vi "Snapshot Viewer.vi"() -> ()   [LabVIEW 2018]
uses:
  <userlib>/Jet Engineering/JET_QSM/Code/Private/JET_QSM - Add State [String API].vi
  <userlib>/Jet Engineering/JET_QSM/Code/Private/JET_QSM_InvalidOption STYP.ctl
  Private/Status STYP.ctl
  Classes/Video File/Video File.lvclass
  Classes/Video Frame/Video Frame.lvclass
  <vilib>/vision/Image Controls.llb/IMAQ Image.ctl
  Classes/Message/Message.lvclass
  Classes/Depth Data Message/Depth Data Message.lvclass
  Classes/STOP Message/STOP.lvclass
  <vilib>/Utility/Data Type/NI_Data Type.lvlib
  C:/Users/aaron.jencks/Documents/GitHub/emerson_seed_object_detection/LabVIEW/Projects/Paul's Video Viewer/Classes/Message/Message.lvclass
  Shared/Roughness Parameters STYP.ctl
panel:
  in  "Clear?":bool
  out "Ready?":bool
  out "Saved Indices":u32[](array[numeric])
  in  "Keep?":bool
  in  "stop":bool
  out "File Opened?":bool
  out "Frame Count":u32
  in  "Frame Index":u32
  out "Roughness Parameters":T1
  in  "Path":path
  out "Image":T2(plugin-control)
  out "Recent states before Error (with tick counts) 2":string="0.167 sec ago: VI Initialize\n0.167 sec ago: Window Open\n0.110 sec ago: Control Update\n0.110 sec ago: Indicator Update\n0.000 sec ago: Error Handler\r\n"
  out "error out":errorcluster
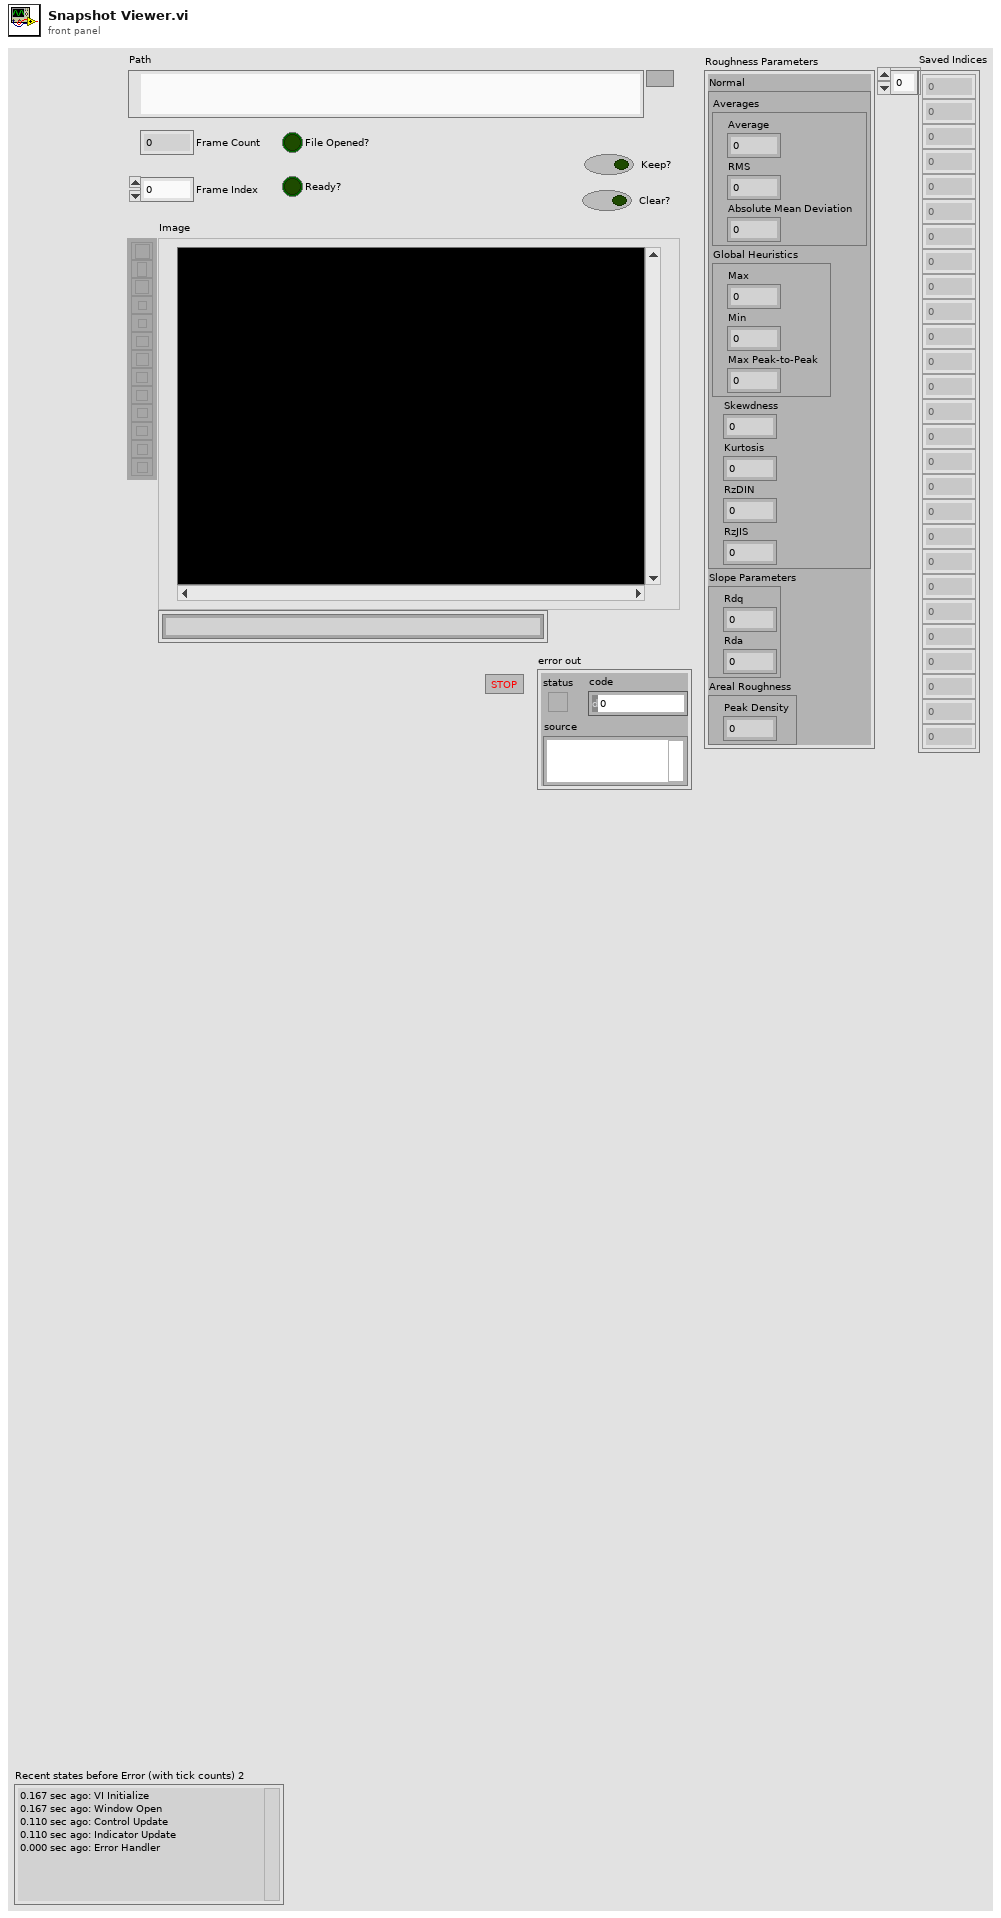
[diagram p1: front panel]
types:
  T1 = typedef "Roughness Parameters STYP.ctl" = cluster{"Normal":cluster{"Averages":cluster{"Average":dbl, "RMS":dbl, "Absolute Mean Deviation":dbl}, "Global Heuristics":cluster{"Max":dbl, "Min":dbl, "Max Peak-to-Peak":dbl}, "Skewdness":dbl, "Kurtosis":dbl, "RzDIN":dbl, "RzJIS":dbl}, "Slope Parameters":cluster{"Rdq":dbl, "Rda":dbl}, "Areal Roughness":cluster{"Peak Density":dbl}}
  T2 = typedef "IMAQ Image.ctl" = refnum<image>
  T3 = typedef "Status STYP.ctl" = cluster{"VI":cluster{"error":errorcluster, "isExiting?":bool}, "UserLoggedIn?":bool, "Frame Index":u32, "Video File":refnum<class "Video File.lvclass">, "Current Frame":refnum<class "Video Frame.lvclass">, "Image Placeholder":T2, "data log queue":refnum<queue>, "stop queue":refnum<queue>, "Saved Indices":u32[], "ready queue":refnum<queue>}
  T4 = typedef "JET_QSM_InvalidOption STYP.ctl" = enum16{"Ignore", "Dialog", "Error"}
  T5 = typedef "JET_QSM_Refnum STYP.ctl" = cluster{"state":cluster{"queue":refnum<queue>, "idle":string, "error":string, "STOP":string}, "debug":cluster{"enabled?":bool, "queue":refnum<queue>}, "Invalid.option":T4, "QSM.Name":string}
  T6 = enum32{"invalid app kind", "Development System", "Run Time System", "Student Edition", "Embedded LabVIEW", "Evaluation", "Custom"}
  T7 = typedef "JET_QSM_Element STYP.ctl" = cluster{"state":string, "data":variant, "comment":string}
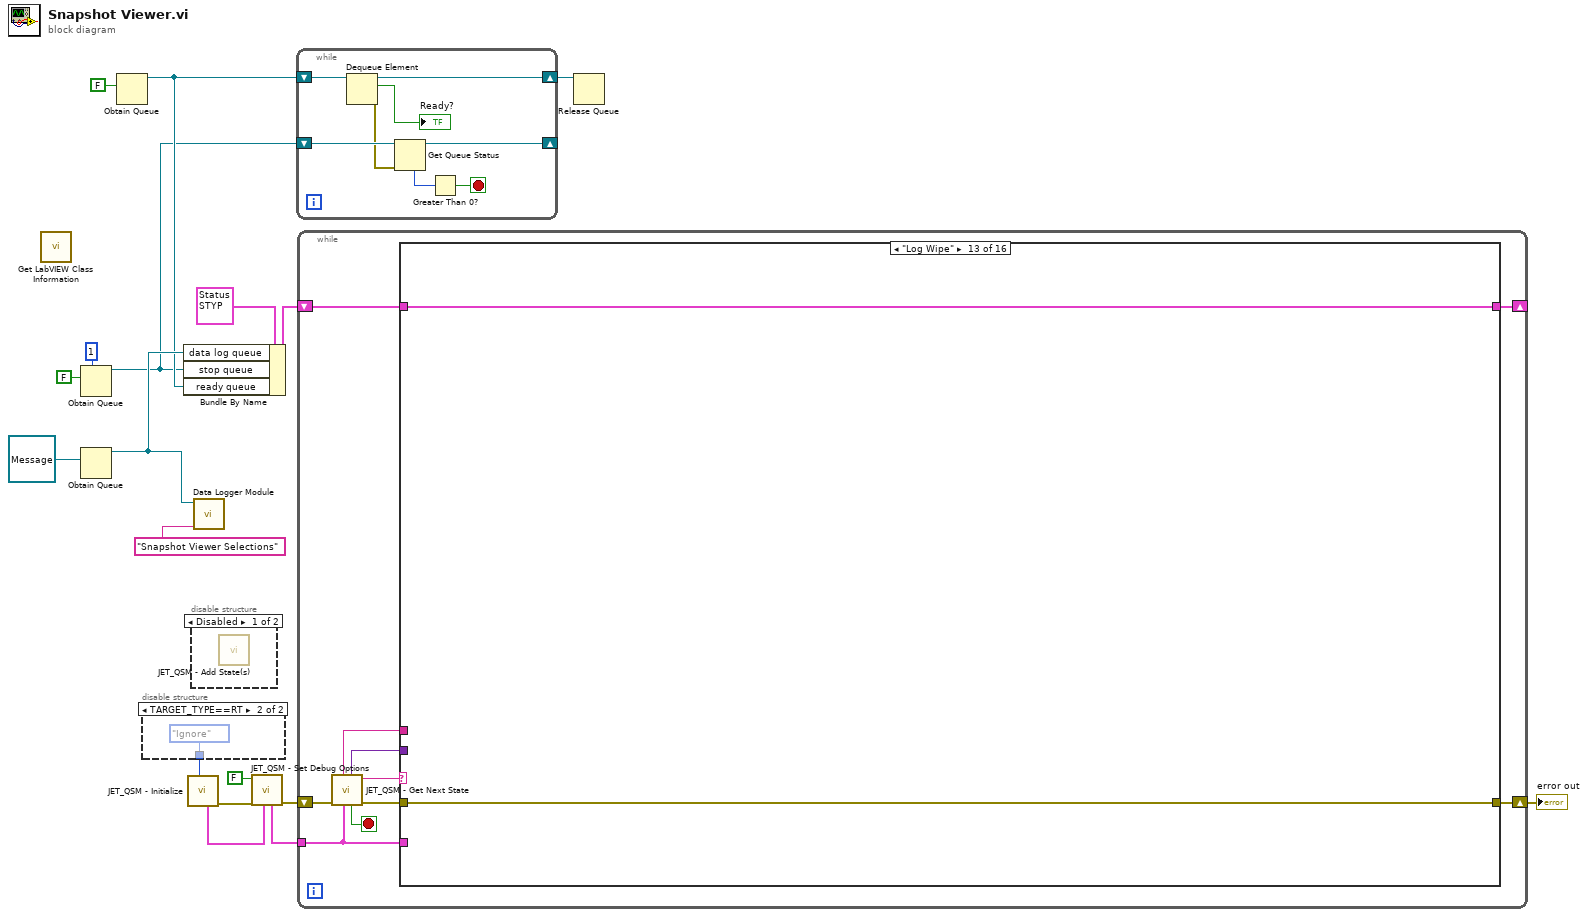
[diagram p0: block diagram]
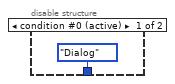
[diagram p2: hidden frame]
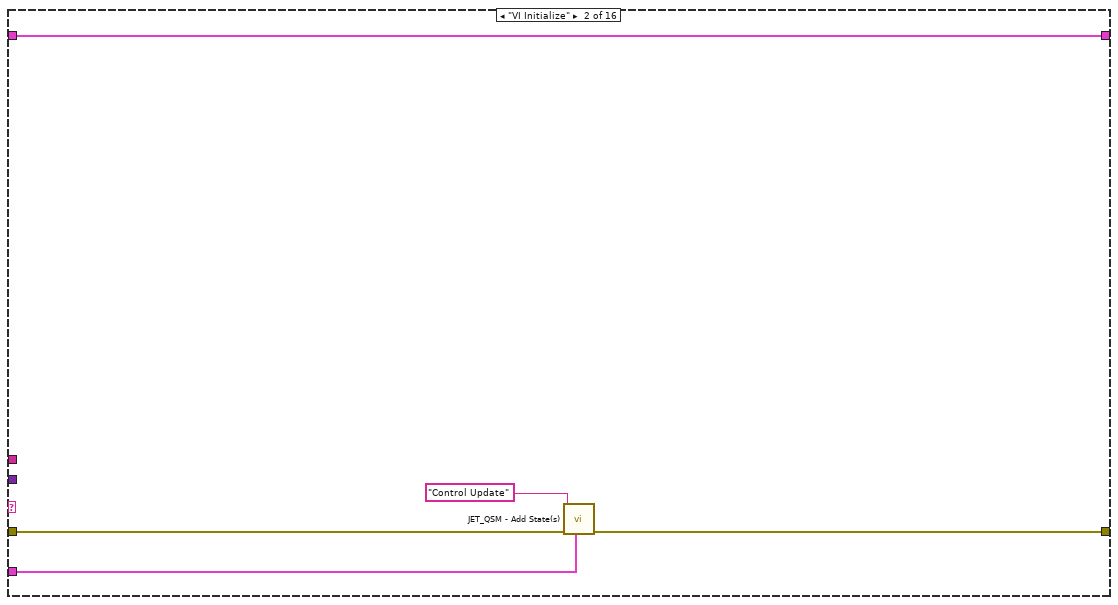
[diagram p5: hidden frame]
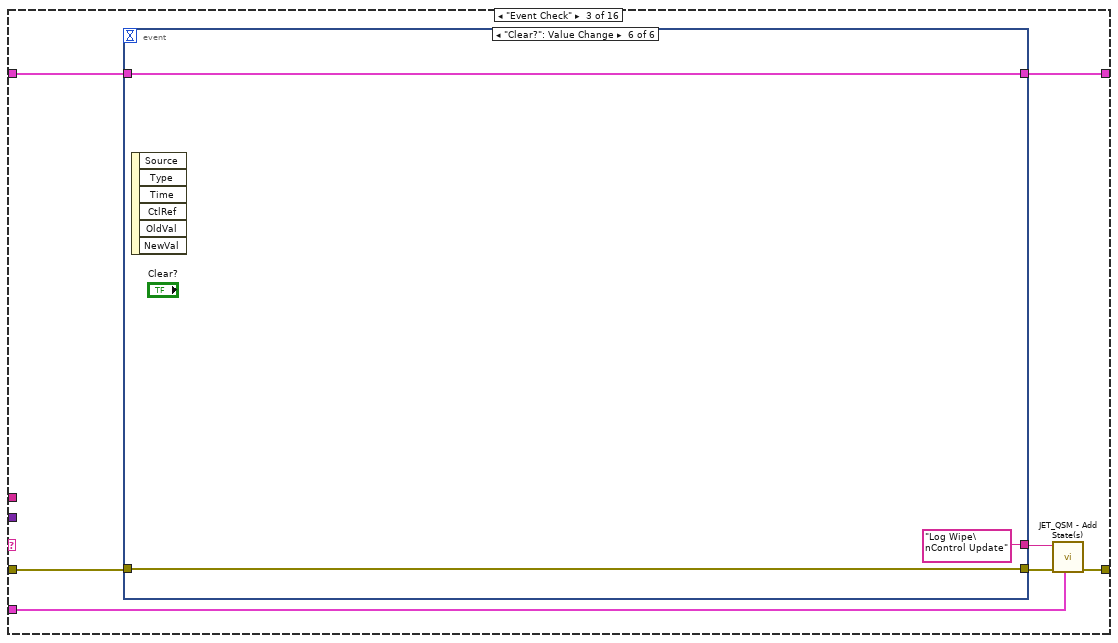
[diagram p6: hidden frame]
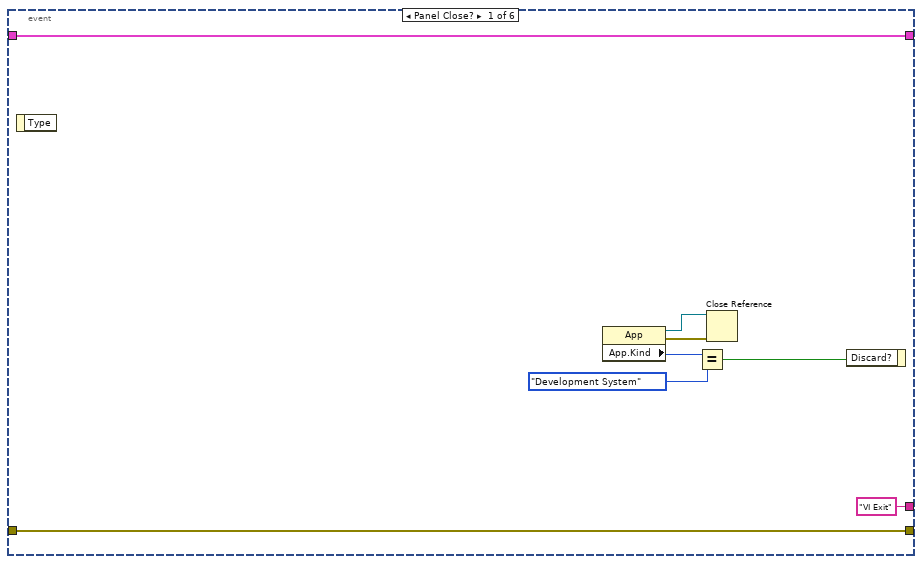
[diagram p7: hidden frame]
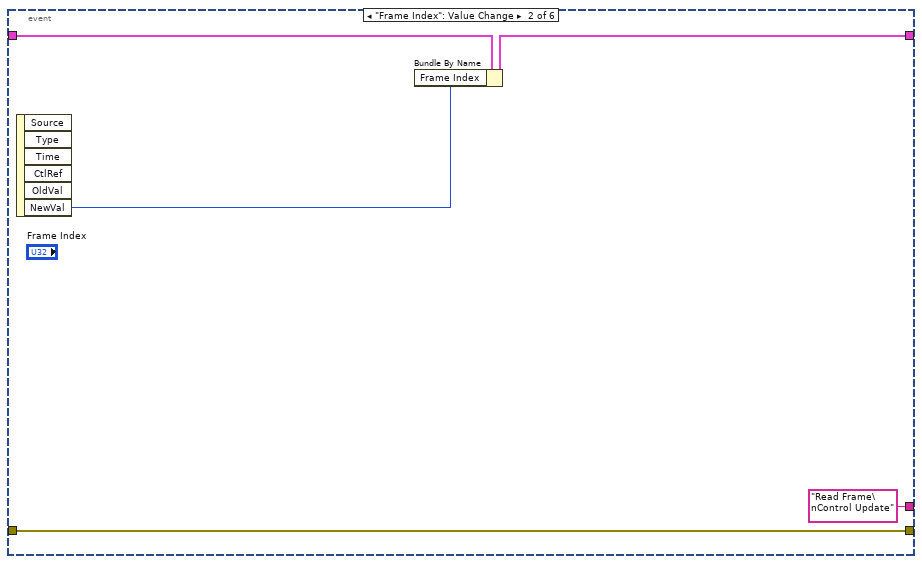
[diagram p8: hidden frame]
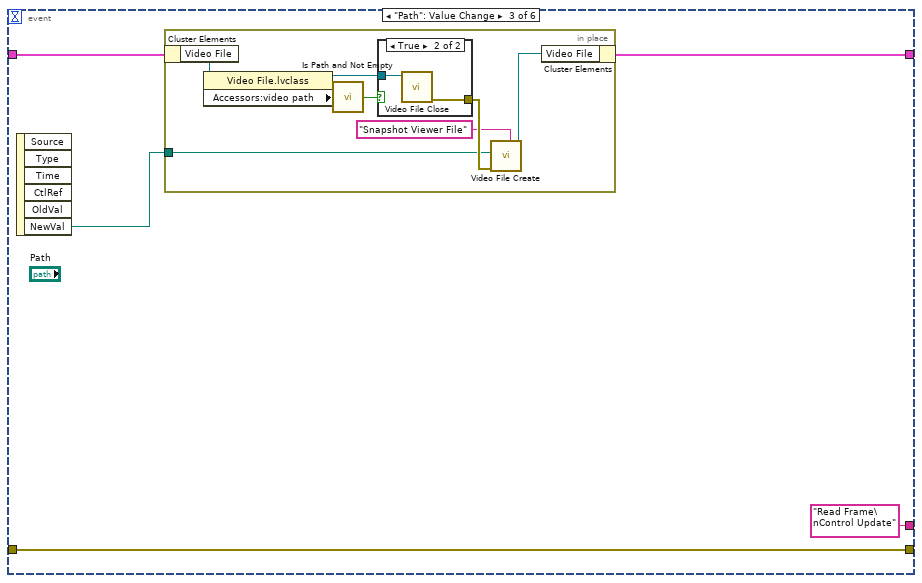
[diagram p9: hidden frame]
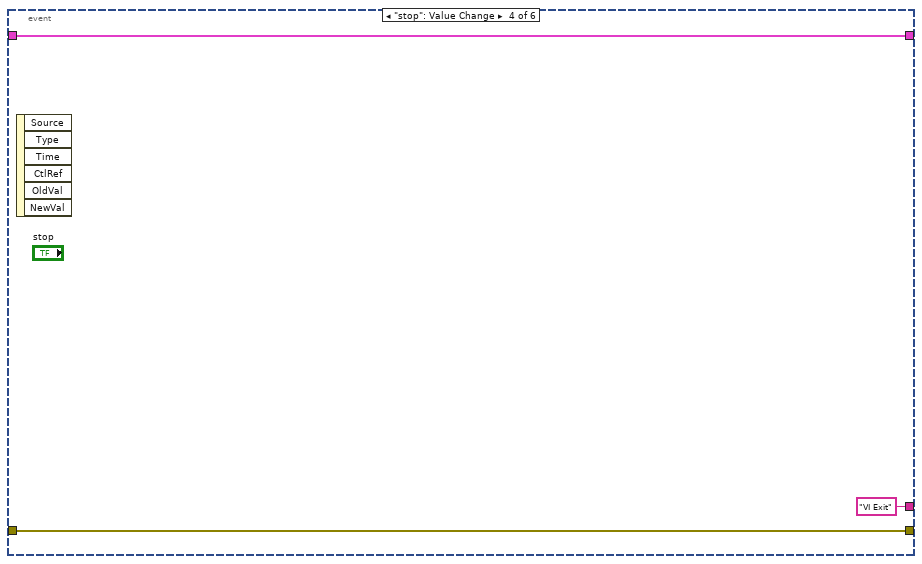
[diagram p11: hidden frame]
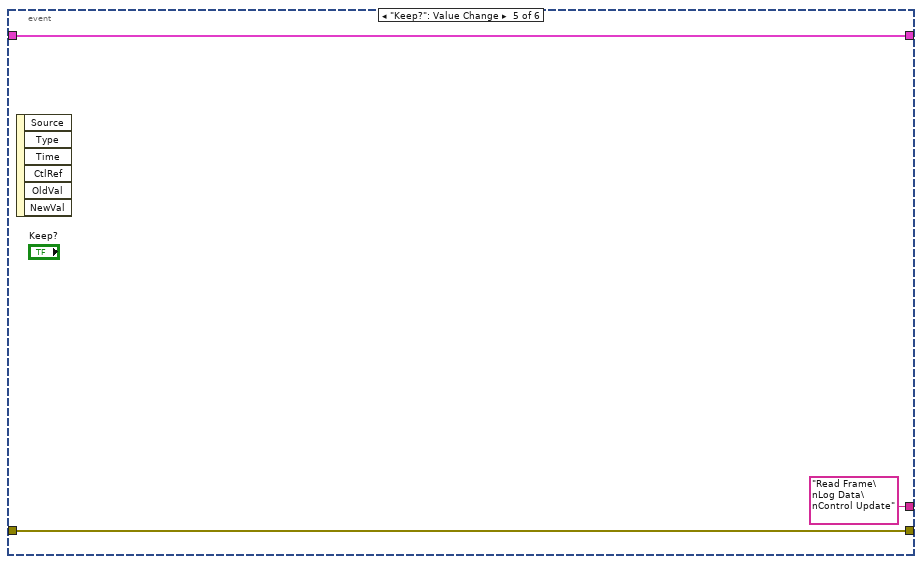
[diagram p12: hidden frame]
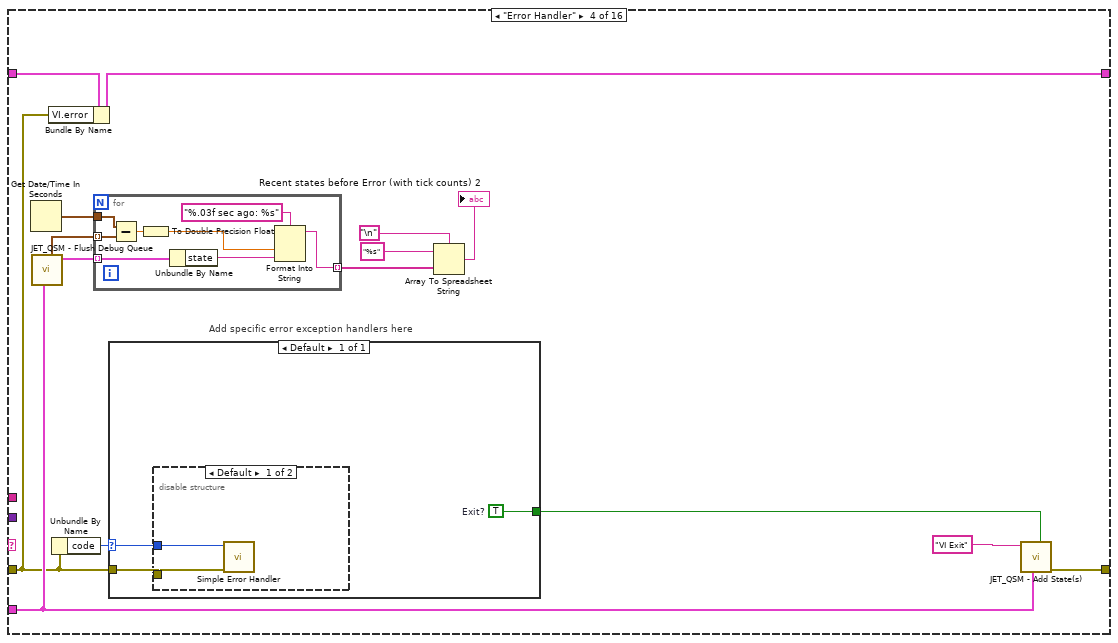
[diagram p13: hidden frame]
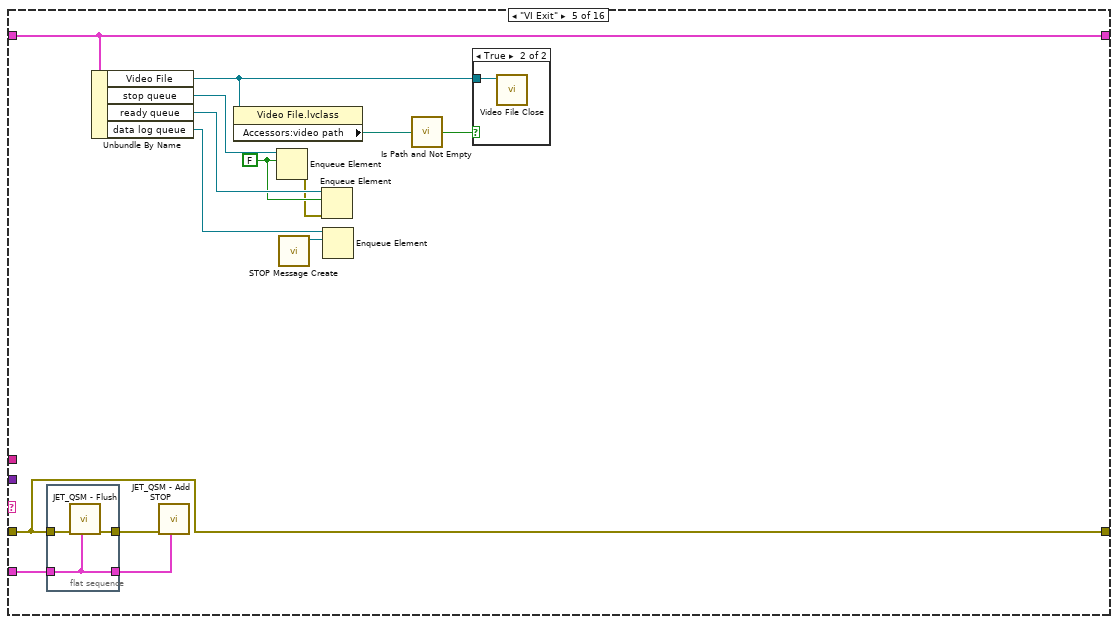
[diagram p15: hidden frame]
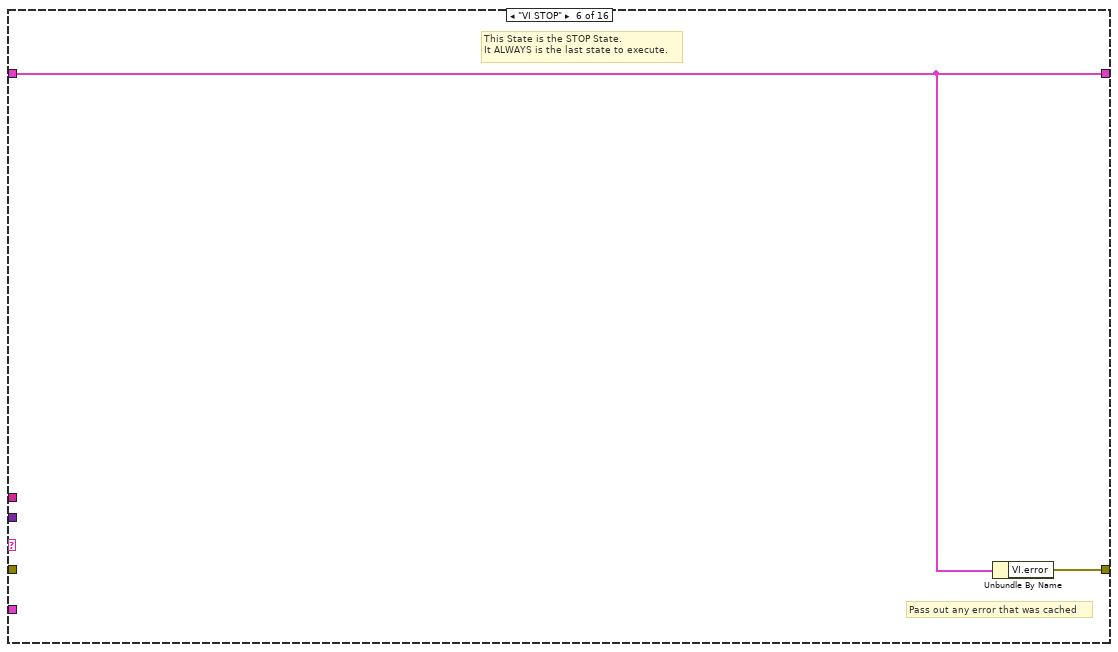
[diagram p17: hidden frame]
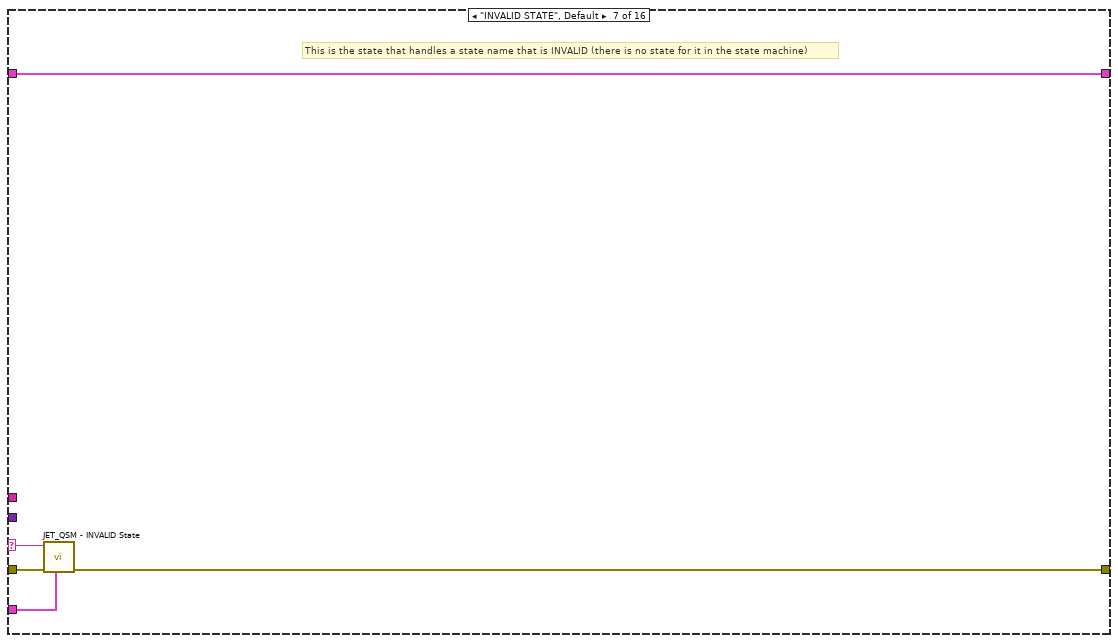
[diagram p18: hidden frame]
diagram:
  n1 = call <vilib>:"Get LabVIEW Class Information.vi"() -> ()  [unwired: 9 in, 3 out]
  n2 = Obtain Queue(max queue size (-1, unlimited)=1, element data type=FALSE) -> (queue out=w3:refnum<queue>)  [unwired: 3 in, 2 out]
  n3 = Obtain Queue(element data type=refnum<class "Message.lvclass"> refnum ("Message.lvclass")) -> (queue out=w7:refnum<queue>)  [unwired: 4 in, 2 out]
  n4 = Obtain Queue(element data type=FALSE) -> (queue out=w4:refnum<queue>)  [unwired: 4 in, 2 out]
  n5 = disable-structure shown="TARGET_TYPE==RT" {
    disable-tunnel: [JET_QSM_InvalidOption_STYP."Dialog" ("invalid state action (Dialog)") JET_QSM_InvalidOption_STYP."Ignore" ("invalid state action (Dialog)")] -> w18
    frame condition #0 (active) {
    }
    frame condition #1 {
    }
  }
  n6 = Bundle By Name(cluster=T3 {"VI"={"error"={"status"=FALSE, "code"=0, "source"=""}, "isExiting?"=FALSE}, "UserLoggedIn?"=FALSE, "Frame Index"=0, "Video File"=refnum, "Current Frame"=refnum, "Image Placeholder"=refnum, "data log queue"=refnum, "stop queue"=refnum, "Saved Indices"=[], "ready queue"=refnum} ("Status"), "data log queue"=w7, "stop queue"=w3, "ready queue"=w4) -> (w8:T3)
  n7 = call <userlib>:"JET_QSM - Initialize.vi"("invalid state action (Dialog)"=w18) -> ("error out"=w12:errorcluster, "Jet_QSM refnum"=w15:T5)  [unwired: 9 in]
  n8 = disable-structure shown="Disabled" {
    frame Disabled {
      n9 = call-poly <userlib>:"JET_QSM - Add State(s).vi"() -> ()  [unwired: 11 in, 1 out]
    }
    frame Enabled {
    }
  }
  n10 = call "Data Logger Module.vi"("Identifier"="Snapshot Viewer Selections", "Message queue"=w7) -> ()  [unwired: 10 in]
  n11 = call <userlib>:"JET_QSM - Set Debug Options.vi"("Jet_QSM refnum"=w15, "error in (no error)"=w12, "debug.enabled? (F)"=FALSE) -> ("error out"=w13:errorcluster, "Jet_QSM ref"=w14:T5)  [unwired: 7 in]
  n12 = while {
    shift-right: [w26] -> w2
    shift-left: w4 -> [w28]
    shift-right: [w22] -> _
    shift-left: w3 -> [w25]
    stop <- w23 stop-if-true
    n13 = Dequeue Element(queue=w28) -> (queue out=w26:refnum<queue>, element=→"Ready?":bool, error out=w21:errorcluster)  [unwired: 2 in, 1 out]
    n14 = Get Queue Status(queue=w25, error in (no error)=w21) -> (queue out=w22:refnum<queue>, # elements in queue=w24:i32)  [unwired: 1 in, 6 out]
    n15 = Greater Than 0?(x=w24) -> (x > 0?=w23:bool)
  }
  n16 = while {
    tunnel: w14 -> [w34]
    shift-right: [w32] -> _
    shift-left: w8 -> [w33]
    shift-right: [w31] -> w17
    shift-left: w13 -> [w38]
    stop <- w35 stop-if-true
    n17 = call <userlib>:"JET_QSM - Get Next State.vi"("Jet_QSM refnum"=w34, "error in (no error)"=w38) -> ("error out"=w37:errorcluster, "state"=w36:string, "Stop Loop?"=w35:bool, "state data"=w30:variant, "state comment"=w29:string)  [unwired: 5 in]
    n18 = case shown="\"Log Wipe\"" w36 {
      selector: w36 -> [_ _ _ _ _ _ w140 _ _ _ _ _ _ _ _ _]
      tunnel: w37 -> [w39 w43 w52 w91 w131 _ w141 w143 w145 w147 w165 w179 w193 w195 w204 w219]
      tunnel: w34 -> [_ w44 w51 w96 w129 _ w139 _ _ _ _ _ _ _ w205 _]
      tunnel: w33 -> [w40 w45 w47 w92 w127 w136 w142 w144 w146 w148 w163 w174 w194 w196 w202 w218]
      tunnel: [w40 w45 w46 w90 w127 w136 w142 w144 w146 w148 w161 w172 w194 w196 w202 w218] -> w32
      tunnel: [w39 w42 w49 w97 w131 w137 w138 w143 w145 w147 w165 w179 w193 w195 w203 w219] -> w31
      tunnel: w30 -> [_ _ _ _ _ _ _ _ _ _ _ _ _ _ _ _]
      tunnel: w29 -> [_ _ _ _ _ _ _ _ _ _ _ _ _ _ _ _]
      frame "------ Standard States ------" {
        # "Standard States are required states for a JET_QSM State Machine\n\nTheir names may be changed; use the Initialize function to specify the new names"
        # "This is a section header; the state is never expected to execute"
      }
      frame "VI Initialize" {
        n19 = call-poly <userlib>:"JET_QSM - Add State(s).vi"("Jet_QSM refnum"=w44, "error in (no error)"=w43, "state(s)"="Control Update") -> ("error out"=w42:errorcluster)  [unwired: 8 in]
      }
      frame "Event Check" {
        n20 = event shown="[5] \"Clear?\": Value Change" {
          selector: _ -> [_ _ _ _ _ _]
          dyn-events: _ -> [_ _ _ _ _ _]
          timeout: _ -> [_ _ _ _ _ _]
          tunnel: w52 -> [w54 w65 w70 w82 w85 w88]
          tunnel: ["VI Exit" ("state(s)") "Read Frame\nControl Update" ("state(s)") "Read Frame\nControl Update" ("state(s)") "VI Exit" ("state(s)") "Read Frame\nLog Data\nControl Update" ("state(s)") "Log Wipe\nControl Update" ("state(s)")] -> w50
          tunnel: [w54 w65 w70 w82 w85 w88] -> w48
          tunnel: w47 -> [w53 w63 w68 w83 w86 w89]
          tunnel: [w53 w61 w67 w83 w86 w89] -> w46
          event Panel Close? {
            n21 = event-data() -> ()  [unwired: 1 in, 1 out]
            n22 = property class="App"() -> (reference out=w56:refnum<vi>, error out=w57:errorcluster, "App.Kind"=w60:T6)  [unwired: 2 in]
            n23 = Equal?(x=w60, y=T6."Development System") -> (x = y?=w58:bool)
            n24 = Close Reference(reference=w56, error in (no error)=w57) -> ()  [unwired: 1 out]
            n25 = event-data("Discard?"=w58) -> ()  [unwired: 1 in, 1 out]
          }
          event "Frame Index": Value Change {
            n26 = event-data() -> ("NewVal"=w62:u32)  [unwired: 1 in, 5 out]
            n27 = Bundle By Name(cluster=w63, "Frame Index"=w62) -> (w61:T3)
          }
          event "Path": Value Change {
            n28 = event-data() -> ("NewVal"=w66:path)  [unwired: 1 in, 5 out]
            n29 = in-place {
              in-place-border: w66 -> [w72]
              n30 = in-place-cluster #1(w68) -> ("Video File"=w78:refnum<class "Video File.lvclass">)
              n31 = property class="Video File.lvclass"(reference=w78) -> (reference out=w75:refnum<class "Video File.lvclass">, "Accessors:video path"=w77:path)  [unwired: 1 in, 1 out]
              n32 = call <vilib>:"Is Path and Not Empty.vi"("path"=w77) -> ("Is Path and Not Empty?"=w76:bool)  [unwired: 4 in]
              n33 = case shown="True" w76 {
                tunnel: w75 -> [_ w80]
                tunnel: [_ w79] -> w73
                frame False {
                }
                frame True {
                  n34 = call-dynamic "Video File Close.vi"("Video File in"=w80) -> ("error out"=w79:errorcluster)  [unwired: 9 in, 1 out]
                }
              }
              n35 = call "Video File Create.vi"("Identifier"="Snapshot Viewer File", "error in (no error)"=w73, "Video Path (\"\")"=w72) -> ("Video File out"=w74:refnum<class "Video File.lvclass">)  [unwired: 7 in, 1 out]
              n36 = in-place-cluster #1("Video File"=w74) -> (w67:T3)
            }
          }
          event "stop": Value Change {
            n37 = event-data() -> ()  [unwired: 1 in, 6 out]
          }
          event "Keep?": Value Change {
            n38 = event-data() -> ()  [unwired: 1 in, 6 out]
          }
          event "Clear?": Value Change {
            n39 = event-data() -> ()  [unwired: 1 in, 6 out]
          }
        }
        n40 = call-poly <userlib>:"JET_QSM - Add State(s).vi"("Jet_QSM refnum"=w51, "error in (no error)"=w48, "state(s)"=w50) -> ("error out"=w49:errorcluster)  [unwired: 8 in]
      }
      frame "Error Handler" {
        # "Add specific error exception handlers here"
        n41 = Get Date/Time In Seconds() -> (seconds since 1Jan1904=w100:timestamp)
        n42 = call <userlib>:"JET_QSM - Flush Debug Queue.vi"("Jet_QSM refnum"=w96) -> ("QSM Elements"=w98:T7[], "Timestamps"=w99:timestamp[])  [unwired: 8 in, 1 out]
        n43 = Bundle By Name(cluster=w92, "VI.error"=w91) -> (w90:T3)
        n44 = Unbundle By Name(w91) -> ("code"=w93:i32)
        n45 = for {
          tunnel: w98 -> [w112] mode=indexing
          tunnel: [w110] -> w102 mode=indexing
          tunnel: w100 -> [w107]
          tunnel: w99 -> [w108] mode=indexing
          n46 = Subtract(x=w107, y=w108) -> (x-y=w106:dbl)
          n47 = To Double Precision Float(number=w106) -> (double precision float=w105:dbl)
          n48 = Unbundle By Name(w112) -> ("state"=w111:string)
          n49 = Format Into String(format string="%.03f sec ago: %s", w105, w111) -> (resulting string=w110:string)  [unwired: 2 in, 1 out]
        }
        n50 = case shown="Default" w93 {
          selector: w93 -> [w114]
          tunnel: [w115] -> w94
          tunnel: w91 -> [w113]
          frame Default {
            w115 = TRUE  # Exit?
            n51 = disable-structure shown="Default" {
              disable-tunnel: w114 -> [w117 _]
              disable-tunnel: w113 -> [w116 _]
              frame condition #0 (active) {
                n52 = call <vilib>:"Simple Error Handler.vi"("error code (no error:0)"=w117, "error in (no error)"=w116) -> ()  [unwired: 3 in, 5 out]
              }
              frame condition #1 {
              }
            }
          }
        }
        n53 = Array To Spreadsheet String(delimiter (Tab)="\n", array=w102, 3:"%s" ("format string")) -> (spreadsheet string=→"Recent states before Error (with tick counts) 2":string)
        n54 = call-poly <userlib>:"JET_QSM - Add State(s).vi"("act? (T)"=w94, "Jet_QSM refnum"=w96, "state(s)"="VI Exit") -> ("error out"=w97:errorcluster)  [unwired: 8 in]
      }
      frame "VI Exit" {
        w121 = FALSE ("element")
        n55 = flat-sequence {
          tunnel: w131 -> [w135]
          tunnel: [w134] -> w130
          tunnel: w129 -> [w133]
          tunnel: [w133] -> w128
          frame #0 {
            n56 = call <userlib>:"JET_QSM - Flush.vi"("Jet_QSM ref"=w133, "error in (no error)"=w135) -> ("error out"=w134:errorcluster)  [unwired: 8 in, 1 out]
          }
        }
        n57 = Unbundle By Name(w127) -> ("Video File"=w124:refnum<class "Video File.lvclass">, "stop queue"=w123:refnum<queue>, "ready queue"=w122:refnum<queue>, "data log queue"=w119:refnum<queue>)
        n58 = call <userlib>:"JET_QSM - Add STOP.vi"("Jet_QSM refnum"=w128, "error in (no error)"=w130) -> ()  [unwired: 9 in, 1 out]
        n59 = property class="Video File.lvclass"(reference=w124) -> ("Accessors:video path"=w126:path)  [unwired: 1 in, 2 out]
        n60 = Enqueue Element(queue=w123, element=w121) -> (error out=w120:errorcluster)  [unwired: 2 in, 2 out]
        n61 = call "STOP Message Create.vi"() -> ("STOP out"=w118:refnum<class "STOP.lvclass">)  [unwired: 10 in, 1 out]
        n62 = Enqueue Element(queue=w122, element=w121, error in (no error)=w120) -> ()  [unwired: 1 in, 3 out]
        n63 = Enqueue Element(queue=w119, element=w118) -> ()  [unwired: 2 in, 3 out]
        n64 = call <vilib>:"Is Path and Not Empty.vi"("path"=w126) -> ("Is Path and Not Empty?"=w125:bool)  [unwired: 4 in]
        n65 = case shown="True" w125 {
          tunnel: w124 -> [_ w132]
          frame False {
          }
          frame True {
            n66 = call-dynamic "Video File Close.vi"("Video File in"=w132) -> ()  [unwired: 9 in, 2 out]
          }
        }
      }
      frame "VI STOP" {
        # "Pass out any error that was cached"
        # "This State is the STOP State.\nIt ALWAYS is the last state to execute."
        n67 = Unbundle By Name(w136) -> ("VI.error"=w137:errorcluster)
      }
      frame "INVALID STATE", Default {
        # "This is the state that handles a state name that is INVALID (there is no state for it in the state machine)"
        n68 = call <userlib>:"JET_QSM - INVALID State.vi"("Jet_QSM refnum"=w139, "error in (no error)"=w141, "state"=w140) -> ("error out"=w138:errorcluster)  [unwired: 8 in]
      }
      frame "------ Menu Commands ------" {
        # "This is a section header; the state is never expected to execute"
      }
      frame "------ Events  ------" {
        # "This is a section header; the state is never expected to execute"
      }
      frame "------ Actions  ------" {
        # "This is a section header; the state is never expected to execute"
      }
      frame "Read Frame" {
        n69 = Unbundle By Name(w163) -> ("Video File"=w157:refnum<class "Video File.lvclass">, "Frame Index"=w155:u32, "Image Placeholder"=w164:T2)
        n70 = property class="Video File.lvclass"(reference=w157) -> ("Accessors:Number of Frames"=w154:u32)  [unwired: 1 in, 2 out]
        n71 = Greater Or Equal?(x=w155, y=w154) -> (x >= y?=w156:bool)
        n72 = Decrement(x=w154) -> (x-1=w153:u32)
        n73 = Select(t=w153, s=w156, f=w155) -> (s? t:f=w151:u32)
        n74 = Less Than 0?(x=w151) -> (x < 0?=w152:bool)
        n75 = Select(t=u32 0, s=w152, f=w151) -> (s? t:f=w149:u32)
        n76 = property class="Video File.lvclass"(reference=w157, "Accessors:Frame Number"=w149) -> (reference out=w160:refnum<class "Video File.lvclass">, "Accessors:video path"=w159:path)  [unwired: 1 in, 1 out]
        n77 = call <vilib>:"Is Path and Not Empty.vi"("path"=w159) -> ("Is Path and Not Empty?"=w158:bool)  [unwired: 4 in]
        n78 = case shown="True" w158 {
          tunnel: w164 -> [_ w168]
          tunnel: [_ w167] -> w162
          tunnel: w160 -> [_ w166]
          frame False {
          }
          frame True {
            n79 = call-dynamic "Video File Frame Read.vi"("Image Dst"=w168, "Video File in"=w166) -> ("Video Frame out"=w167:refnum<class "Video Frame.lvclass">)  [unwired: 5 in, 4 out]
          }
        }
        n80 = Bundle By Name(cluster=w163, "Current Frame"=w162) -> (w161:T3)
      }
      frame "Log Data" {
        n81 = Unbundle By Name(w174) -> ("Saved Indices"=w176:u32[], "Frame Index"=w175:u32, "Current Frame"=w178:refnum<class "Video Frame.lvclass">, "data log queue"=w177:refnum<queue>, "ready queue"=w170:refnum<queue>)
        n82 = flat-sequence {
          tunnel: w178 -> [w189]
          tunnel: w177 -> [w188]
          tunnel: w176 -> [w187]
          tunnel: w175 -> [w186]
          tunnel: [w185] -> w171
          tunnel: w170 -> [w184]
          tunnel: [w182] -> w169
          tunnel: [w192] -> w173
          tunnel: w171 -> [w192]
          tunnel: w169 -> [w191]
          frame #0 {
            n83 = call "Compute Roughness Params.vi"("Video Frame"=w189) -> ("Roughness Parameters"=w181:T1)  [unwired: 4 in]
            n84 = call "Depth Data Message Create.vi"("Roughness"=w181) -> ("Depth Data Message out"=w180:refnum<class "Depth Data Message.lvclass">)  [unwired: 9 in, 1 out]
            n85 = Build Array (concatenate)(w187, w186) -> (w185:u32[])
            n86 = Enqueue Element(queue=w184, element=FALSE) -> (queue out=w182:refnum<queue>)  [unwired: 2 in, 2 out]
            n87 = Enqueue Element(queue=w188, element=w180) -> ()  [unwired: 2 in, 3 out]
          }
          frame #1 {
            n88 = Enqueue Element(queue=w191, element=TRUE) -> ()  [unwired: 2 in, 3 out]
          }
        }
        n89 = Bundle By Name(cluster=w174, "Saved Indices"=w173) -> (w172:T3)
      }
      frame "Log Wipe" {
      }
      frame "------ Window and Panel Control ------" {
        # "This is a section header; the state is never expected to execute"
      }
      frame "Control Update" {
        # "Update all control properties here from the status cluster\n(Consolidate/reduce property nodes)"
        n90 = Unbundle By Name(w202) -> ("Video File"=w201:refnum<class "Video File.lvclass">, "Frame Index"=w200:u32)
        n91 = property class="Video File.lvclass"(reference=w201) -> ("Accessors:video path"=w197:path)  [unwired: 1 in, 2 out]
        n92 = Empty String/Path?(string/path=w197) -> (empty?=w198:bool)
        n93 = call <userlib>:"VI Control - Disable Control.vi"("Disable? (T)"=w198) -> ("Disabled Attribute"=w199:u8)  [unwired: 7 in, 1 out]
        n94 = local write "Path"(w197) -> ()
        n95 = local write "Frame Index"(w200) -> ()
        n96 = property on="Keep?" class="Bool"("DisabledEnum"=w199) -> ()  [unwired: 2 in, 2 out]
        n97 = call-poly <userlib>:"JET_QSM - Add State(s).vi"("Jet_QSM refnum"=w205, "error in (no error)"=w204, "state(s)"="Indicator Update") -> ("error out"=w203:errorcluster)  [unwired: 8 in]
      }
      frame "Indicator Update" {
        # "Update all indicator values here from the status cluster\n(Eliminate Local Variables)"
        n98 = Unbundle By Name(w218) -> ("Video File"=w217:refnum<class "Video File.lvclass">, "Current Frame"=w213:refnum<class "Video Frame.lvclass">, "Saved Indices"=→"Saved Indices":u32[], "ready queue"=w209:refnum<queue>)
        n99 = property class="Video Frame.lvclass"(reference=w213) -> ("Accessors:Image"=→"Image":T2)  [unwired: 1 in, 2 out]
        n100 = property class="Video File.lvclass"(reference=w217) -> ("Accessors:video path"=w216:path, "Accessors:Number of Frames"=→"Frame Count":u32)  [unwired: 1 in, 2 out]
        n101 = call <vilib>:"Is Path and Not Empty.vi"("path"=w216) -> ("Is Path and Not Empty?"=w210:bool)  [unwired: 4 in]
        "File Opened?" <- w210
        n102 = case shown="False" w210 {
          tunnel: w213 -> [_ w225]
          tunnel: [_ w224] -> w212
          tunnel: w209 -> [w220 w223]
          tunnel: [w220 w222] -> w208
          frame False {
          }
          frame True {
            n103 = call "Compute Roughness Params.vi"("Video Frame"=w225) -> ("Roughness Parameters"=w224:T1)  [unwired: 4 in]
            n104 = Enqueue Element(queue=w223, element=FALSE) -> (queue out=w222:refnum<queue>)  [unwired: 2 in, 2 out]
          }
        }
        "Roughness Parameters" <- w212
        n105 = Enqueue Element(queue=w208, element=TRUE) -> ()  [unwired: 2 in, 3 out]
      }
    }
  }
  "error out" <- w17
  n106 = Release Queue(queue=w2) -> ()  [unwired: 2 in, 3 out]
